vi "Time Stamp to String.vi"(8 "error in (no error)":errorcluster, 9 "24 Hr?":bool, 10 "Date Format":string(combo)="%d-%b-%Y", 11 "Time Stamp (Optional)":timestamp) -> (0 "error out":errorcluster, 3 "Output String":string)   [LabVIEW 2016, in "SLL String.lvlib"]
doc: "Converts Time Stamp to String in a format that can be used as part of file names.\n\nIf Time Stamp is not wired, the VI takes the current time and converts it."
uses:
  SLL String.lvlib
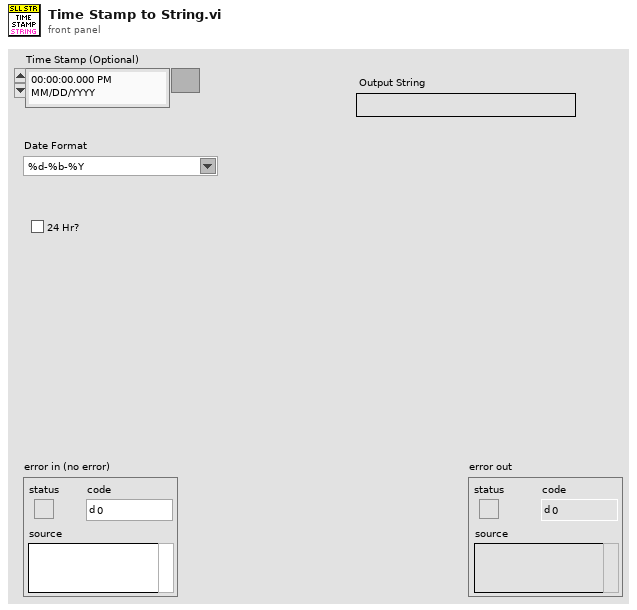
[diagram p1: front panel]
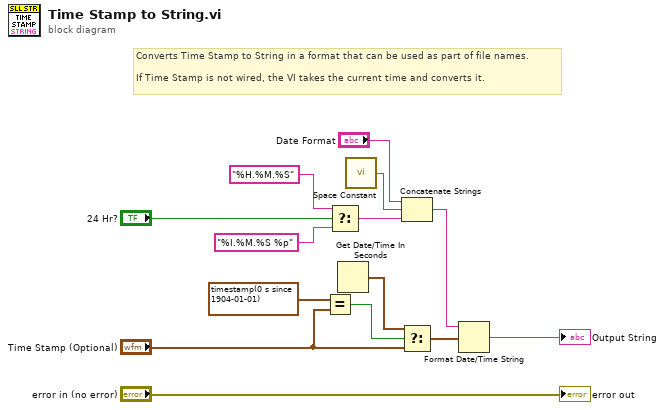
[diagram p0: block diagram]
diagram:
  # "Converts Time Stamp to String in a format that can be used as part of file names.\n\nIf Time Stamp is not wired, the VI takes the current time and converts it."
  n1 = Equal?(x=timestamp(0 s since 1904-01-01), y="Time Stamp (Optional)") -> (x = y?=w4:bool)
  n2 = Select(t="%H.%M.%S" ("time format string (%c)"), s="24 Hr?", f="%I.%M.%S %p" ("time format string (%c)")) -> (s? t:f=w8:string)
  n3 = Get Date/Time In Seconds() -> (seconds since 1Jan1904=w3:timestamp)
  n4 = call <vilib>:"Space Constant.vi"() -> ("String"=w7:string)
  n5 = Concatenate Strings("Date Format", w7, w8) -> (w6:string)
  n6 = Select(t=w3, s=w4, f="Time Stamp (Optional)") -> (s? t:f=w1:timestamp)
  n7 = Format Date/Time String(time format string (%c)=w6, seconds (now)=w1) -> (date/time string=→"Output String":string)  [unwired: 1 in]
  "error out" <- "error in (no error)"
